vi "SP Coerce to Available Formats.vi"(7 "Formatted Data?":bool, 9 "Parameters Measured":T1[](array[typedef]) {"Channel" min=1 max=99 step=1; "Parameter"."Stimulus Port" min=1 step=1; "Parameter"."Response Port" min=1 step=1}, 10 "CH Format":refnum<vi>[](array[refnum]), 11 "CH Measure":refnum<vi>[](array[refnum])) -> ()   [LabVIEW 2011]
uses:
  TypeDefs/SP Parameter to Measure.ctl
  TypeDefs/SP Parameter.ctl
  TypeDefs/SP Calibration State.ctl
  TypeDefs/SP Measurement Format.ctl
  TypeDefs/SP Display Format.ctl
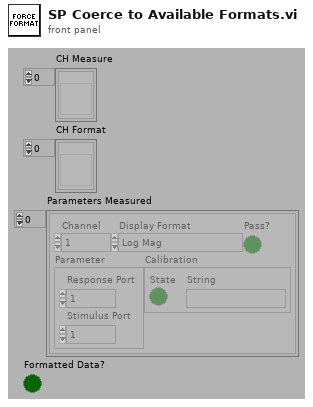
[diagram p1: front panel]
types:
  T1 = typedef "SP Parameter to Measure.ctl" = cluster{"Channel":i8, "Parameter":T2, "Calibration":T3, "Display Format":T4, "Pass?":bool}
  T2 = typedef "SP Parameter.ctl" = cluster{"Stimulus Port":i8, "Response Port":i8}
  T3 = typedef "SP Calibration State.ctl" = cluster{"State":bool, "String":string}
  T4 = typedef "SP Measurement Format.ctl" = enum32{"Log Mag", "Phase", "Delay", "Smith (R+jX)", "Polar (Re/Im)", "Linear Mag", "SWR", "Real", "Imaginary", "Smith (Lin/Phase)", "Smith (Log/Phase)", "Smith (Real/Imag)", "Smith (G+jB)", "Polar (Lin/Phase)", "Polar (Log/Phase)", "Expanded Phase", "Positive Phase", "Inverted Smith", "Unwrapped Phase", "Power Out", "Power In", "Linear Mag/Phase", "Log Mag/Phase", "Real/Imaginary"}
  T5 = typedef "SP Display Format.ctl" = i32
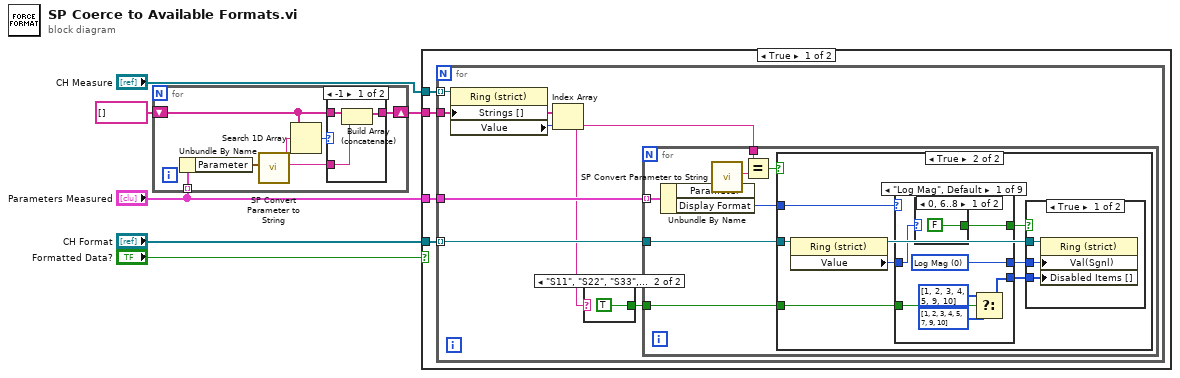
[diagram p0: block diagram]
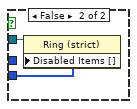
[diagram p5: hidden frame]
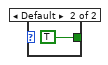
[diagram p6: hidden frame]
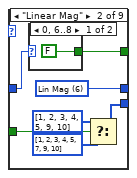
[diagram p7: hidden frame]
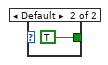
[diagram p8: hidden frame]
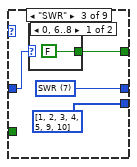
[diagram p9: hidden frame]
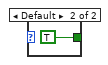
[diagram p10: hidden frame]
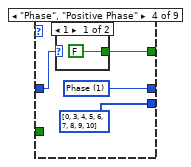
[diagram p11: hidden frame]
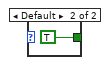
[diagram p12: hidden frame]
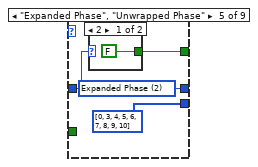
[diagram p13: hidden frame]
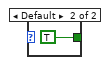
[diagram p14: hidden frame]
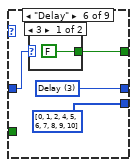
[diagram p15: hidden frame]
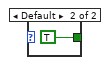
[diagram p16: hidden frame]
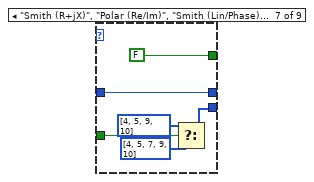
[diagram p17: hidden frame]
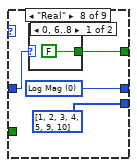
[diagram p18: hidden frame]
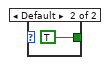
[diagram p19: hidden frame]
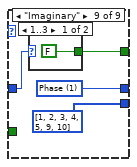
[diagram p20: hidden frame]
diagram:
  n1 = for {
    tunnel: "Parameters Measured" -> [w12] mode=indexing
    shift-right: [w11] -> w1
    shift-left: string[] [] -> [w9]
    n2 = Unbundle By Name(w12) -> ("Parameter"=w10:T2)
    n3 = call "SP Convert Parameter to String.vi"("Parameter"=w10) -> ("Parameter String"=w7:string)  [unwired: 10 out]
    n4 = Search 1D Array(1D array=w9, element=w7) -> (index of element=w8:i32)  [unwired: 1 out]
    n5 = case shown="-1" w8 {
      tunnel: w9 -> [w15 w16]
      tunnel: [w14 w16] -> w11
      tunnel: w7 -> [w13 _]
      frame -1 {
        n6 = Build Array (concatenate)(w15, w13) -> (w14:string[])
      }
      frame Default {
      }
    }
  }
  n7 = case shown="True" "Formatted Data?" {
    tunnel: "Parameters Measured" -> [w20 _]
    tunnel: "CH Measure" -> [w19 w111]
    tunnel: "CH Format" -> [w18 _]
    tunnel: w1 -> [w17 w110]
    frame True {
      n8 = for {
        tunnel: w19 -> [w27] mode=indexing
        tunnel: w20 -> [w26]
        tunnel: w18 -> [w25] mode=indexing
        tunnel: w17 -> [w23]
        n9 = property class="Ring (strict)"(reference=w27, "Strings []"=w23) -> ("Value"=w24:i32)  [unwired: 1 in, 2 out]
        n10 = Index Array(array=w23, index=w24) -> (element=w22:string)
        n11 = case shown="\"S11\", \"S22\", \"S33\", \"S44\", \"S55\", \"S66\", \"S77\", \"S88\"" w22 {
          tunnel: [_ TRUE] -> w21
          frame Default {
          }
          frame "S11", "S22", "S33", "S44", "S55", "S66", "S77", "S88" {
          }
        }
        n12 = for {
          tunnel: w26 -> [w36] mode=indexing
          tunnel: w22 -> [w35]
          tunnel: w25 -> [w32]
          tunnel: w21 -> [w31]
          n13 = Unbundle By Name(w36) -> ("Parameter"=w29:T2, "Display Format"=w33:T4)
          n14 = call "SP Convert Parameter to String.vi"("Parameter"=w29) -> ("Parameter String"=w30:string)  [unwired: 10 out]
          n15 = Equal?(x=w35, y=w30) -> (x = y?=w34:bool)
          n16 = case shown="True" w34 {
            tunnel: w33 -> [_ w44]
            tunnel: w32 -> [_ w42]
            tunnel: w31 -> [_ w37]
            frame False {
            }
            frame True {
              n17 = property class="Ring (strict)"(reference=w42) -> (reference out=w41:refnum<vi>, "Value"=w40:i32)  [unwired: 1 in, 1 out]
              n18 = case shown="\"Log Mag\", Default" w44 {
                tunnel: [w56 w65 w71 w77 w80 w89 w96 w101 w107] -> w43
                tunnel: w40 -> [w55 w64 w70 w76 w83 w88 w96 w100 w106]
                tunnel: [w54 w63 w69 w75 w82 w87 FALSE w99 w105] -> w39
                tunnel: [w51 w60 i32[] [1, 2, 3, 4, 5, 9, 10] ("Disabled Items []") i32[] [0, 3, 4, 5, 6, 7, 8, 9, 10] ("Disabled Items []") i32[] [0, 3, 4, 5, 6, 7, 8, 9, 10] ("Disabled Items []") i32[] [0, 1, 2, 4, 5, 6, 7, 8, 9, 10] ("Disabled Items []") w94 i32[] [1, 2, 3, 4, 5, 9, 10] ("Disabled Items []") i32[] [1, 2, 3, 4, 5, 9, 10] ("Disabled Items []")] -> w38
                tunnel: w37 -> [w50 w59 _ _ _ _ w92 _ _]
                frame "Log Mag", Default {
                  w56 = T5 0 items=["Log Mag", "Phase", "Expanded Phase", "Delay", "Smith", "Polar", "Lin Mag", "SWR", "Loss", "Real", "Imaginary"] ("Format")
                  n19 = case shown="0, 6..8" w55 {
                    tunnel: [FALSE TRUE] -> w54
                    frame 0, 6..8 {
                    }
                    frame Default {
                    }
                  }
                  n20 = Select(t=i32[] [1, 2, 3, 4, 5, 9, 10] ("Disabled Items []"), s=w50, f=i32[] [1, 2, 3, 4, 5, 7, 9, 10] ("Disabled Items []")) -> (s? t:f=w51:i32[])
                }
                frame "Linear Mag" {
                  w65 = T5 6 items=["Log Mag", "Phase", "Expanded Phase", "Delay", "Smith", "Polar", "Lin Mag", "SWR", "Loss", "Real", "Imaginary"] ("Format")
                  n21 = case shown="0, 6..8" w64 {
                    tunnel: [FALSE TRUE] -> w63
                    frame 0, 6..8 {
                    }
                    frame Default {
                    }
                  }
                  n22 = Select(t=i32[] [1, 2, 3, 4, 5, 9, 10] ("Disabled Items []"), s=w59, f=i32[] [1, 2, 3, 4, 5, 7, 9, 10] ("Disabled Items []")) -> (s? t:f=w60:i32[])
                }
                frame "SWR" {
                  w71 = T5 7 items=["Log Mag", "Phase", "Expanded Phase", "Delay", "Smith", "Polar", "Lin Mag", "SWR", "Loss", "Real", "Imaginary"] ("Format")
                  n23 = case shown="0, 6..8" w70 {
                    tunnel: [FALSE TRUE] -> w69
                    frame 0, 6..8 {
                    }
                    frame Default {
                    }
                  }
                }
                frame "Phase", "Positive Phase" {
                  w77 = T5 1 items=["Log Mag", "Phase", "Expanded Phase", "Delay", "Smith", "Polar", "Lin Mag", "SWR", "Loss", "Real", "Imaginary"] ("Format")
                  n24 = case shown="1" w76 {
                    tunnel: [FALSE TRUE] -> w75
                    frame 1 {
                    }
                    frame Default {
                    }
                  }
                }
                frame "Expanded Phase", "Unwrapped Phase" {
                  w80 = T5 2 items=["Log Mag", "Phase", "Expanded Phase", "Delay", "Smith", "Polar", "Lin Mag", "SWR", "Loss", "Real", "Imaginary"] ("Format")
                  n25 = case shown="2" w83 {
                    tunnel: [FALSE TRUE] -> w82
                    frame 2 {
                    }
                    frame Default {
                    }
                  }
                }
                frame "Delay" {
                  w89 = T5 3 items=["Log Mag", "Phase", "Expanded Phase", "Delay", "Smith", "Polar", "Lin Mag", "SWR", "Loss", "Real", "Imaginary"] ("Format")
                  n26 = case shown="3" w88 {
                    tunnel: [FALSE TRUE] -> w87
                    frame 3 {
                    }
                    frame Default {
                    }
                  }
                }
                frame "Smith (R+jX)", "Polar (Re/Im)", "Smith (Lin/Phase)".."Polar (Log/Phase)", "Inverted Smith", "Power Out" {
                  n27 = Select(t=i32[] [4, 5, 9, 10] ("Disabled Items []"), s=w92, f=i32[] [4, 5, 7, 9, 10] ("Disabled Items []")) -> (s? t:f=w94:i32[])
                }
                frame "Real" {
                  w101 = T5 0 items=["Log Mag", "Phase", "Expanded Phase", "Delay", "Smith", "Polar", "Lin Mag", "SWR", "Loss", "Real", "Imaginary"] ("Format")
                  n28 = case shown="0, 6..8" w100 {
                    tunnel: [FALSE TRUE] -> w99
                    frame 0, 6..8 {
                    }
                    frame Default {
                    }
                  }
                }
                frame "Imaginary" {
                  w107 = T5 1 items=["Log Mag", "Phase", "Expanded Phase", "Delay", "Smith", "Polar", "Lin Mag", "SWR", "Loss", "Real", "Imaginary"] ("Format")
                  n29 = case shown="1..3" w106 {
                    tunnel: [FALSE TRUE] -> w105
                    frame 1..3 {
                    }
                    frame Default {
                    }
                  }
                }
              }
              n30 = case shown="True" w39 {
                tunnel: w43 -> [w47 _]
                tunnel: w41 -> [w46 w49]
                tunnel: w38 -> [w45 w48]
                frame True {
                  n31 = property class="Ring (strict)"(reference=w46, "Val(Sgnl)"=w47, "Disabled Items []"=w45) -> ()  [unwired: 1 in, 2 out]
                }
                frame False {
                  n32 = property class="Ring (strict)"(reference=w49, "Disabled Items []"=w48) -> ()  [unwired: 1 in, 2 out]
                }
              }
            }
          }
        }
      }
    }
    frame False {
      n33 = for {
        tunnel: w111 -> [w113] mode=indexing
        tunnel: w110 -> [w112]
        n34 = property class="Ring (strict)"(reference=w113, "Strings []"=w112) -> ()  [unwired: 1 in, 2 out]
      }
    }
  }
